vi "Callback Change Metadata.vi"(6 "Variant":variant, 8 "error in (no error)":errorcluster, 9 "Old Values":string[][](array[string]), 10 "object ref in":T1, 11 "Table Change":T2) -> (0 "error out":errorcluster)   [LabVIEW 2014, in "DAQmx Module Editor Node.lvclass"]
doc: "This VI gets called automatically when changes are made to the 'Channel Direction' column of the table and must handle changes appropriately. Register this callback using the appropriate 'Define Column' VI from the Table API."
uses:
  DAQmx Module Editor Node.lvclass
  <vilib>/NI/DCAF/Tag Editor Core/Table API/Table Manager/Cell Change.ctl
  <vilib>/NI/DCAF/Tag Editor Core/Table API/Table Manager/object ref.ctl
  <vilib>/NI/DCAF/Tag Editor Core/Configuration Editor/Classes/Engine Parent/Engine Parent Editor Node.lvclass
  <vilib>/NI/DCAF/Tag Editor Core/Configuration Editor/Classes/Module editor node/module editor node.lvclass
  module/configuration/DAQmx Module Configuration.lvclass
  module/configuration/DAQmx Module Configuration.lvclass/DAQmx Module Configuration.ctl
  <vilib>/NI/Tag Bus/tag/tag descriptor.lvclass/tag descriptor.ctl
  module/configuration/Get Line Name.vi
  <vilib>/NI/Tag Bus Module Framework/module configuration/FindDuplicate.vi
  <vilib>/Utility/error.llb/Error Cluster From Error Code.vi
  <vilib>/NI/Tag Bus Module Framework/channel/TBM channel.lvclass
  <vilib>/NI/Tag Bus/tag/tag descriptor.lvclass
  <vilib>/NI/DCAF/Tag Editor Core/Table API/Table Manager.lvlib
  <vilib>/NI/DCAF/Tag Editor Core/Table API/Table Manager/Table Manager.lvclass
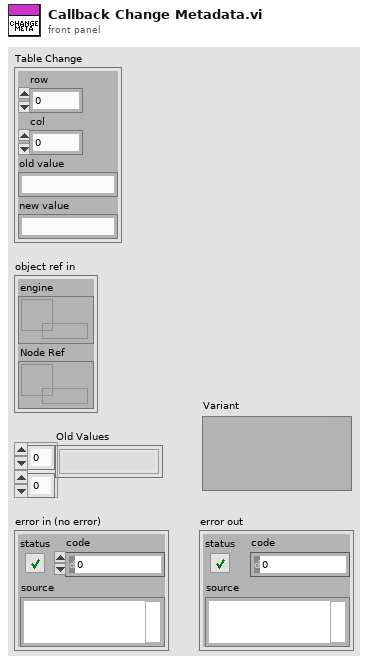
[diagram p1: front panel]
types:
  T1 = typedef "Table Manager.lvlib/Table Manager.lvclass/object ref.ctl" = cluster{"engine":refnum<data-value>, "Node Ref":refnum<data-value>}
  T2 = typedef "Table Manager.lvlib/Cell Change.ctl" = cluster{"row":i32, "col":i32, "old value":string, "new value":string}
  T3 = typedef "DAQmx Module Configuration.lvclass/Line.ctl" = cluster{"channel":refnum<class "TBM channel.lvclass">, "Physical Channel":string, "Measurement Type":T4, "Parameters":T5}
  T4 = typedef "DAQmx Module Configuration.lvclass/Measurement Type.ctl" = enum16{"Digital Input", "Digital Output", "Voltage Input", "Voltage Output", "Current Input", "Current Output", "RTD", "Thermocouple", "Strain"}
  T5 = typedef "DAQmx Module Configuration.lvclass/Parameters.ctl" = cluster{"Digital Config":cluster{"Invert Lines?":bool}, "Voltage Config":cluster{"Maximum Value (V)":dbl, "Minimum Value (V)":dbl, "in terminal configuration (V)":i32, "out terminal configuration (V)":i32}, "Current Config":cluster{"Maximum Value (A)":dbl, "Minimum Value (A)":dbl, "shunt resistor location":i32, "input terminal configuration (C)":i32, "external shunt resistor value":dbl}, "RTD Config":cluster{"Maximum Value (°C)":dbl, "Minimum Value (°C)":dbl, "resistance configuration":i32, "r0":dbl, "current excitation value":dbl, "rtd type":i32, "current excitation source":i32}, "Thermocouple Config":cluster{"Minimum Value (C)":dbl, "Maximum Value (C)":dbl, "thermocouple type":i32, "cjc source":i32, "cjc value":dbl}, "Strain Config":cluster{"Maximum Value":dbl, "Minimum Value":dbl, "bridge information":cluster{"strain configuration":i32, "lead wire resistance":dbl, "initial bridge voltage":dbl, "voltage excitation source":i32, "voltage excitation value":dbl}, "strain gage information":cluster{"gage factor":dbl, "nominal gage resistance":dbl, "poisson ratio":dbl}}}
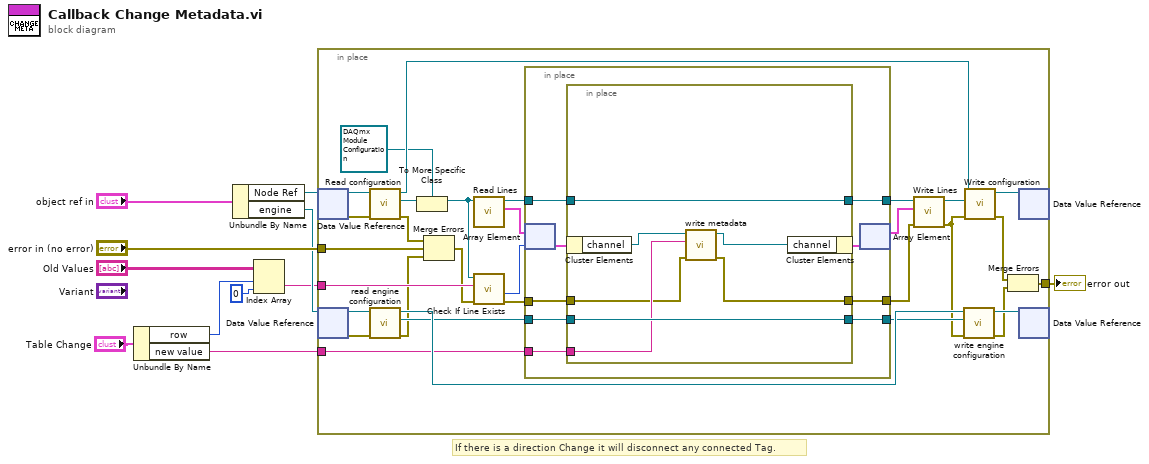
[diagram p0: block diagram]
diagram:
  # "If there is a direction Change it will disconnect any connected Tag."
  n1 = Unbundle By Name("Table Change") -> ("row"=w2:i32, "new value"=w1:string)
  n2 = Unbundle By Name("object ref in") -> ("Node Ref"=w8:refnum<data-value>, "engine"=w7:refnum<data-value>)
  n3 = Index Array(array="Old Values", index (row)=w2, index (col)=0 ("disabled index (col)")) -> (element=w3:string)
  n4 = in-place {
    in-place-border: [w35] -> w11
    in-place-border: "error in (no error)" -> [w13]
    in-place-border: w1 -> [w23]
    in-place-border: w3 -> [w22]
    n5 = in-place-dvr #1(w8) -> (w32:refnum<class "module editor node.lvclass">, w34:errorcluster)
    n6 = in-place-dvr #2(w7) -> (w41:refnum<class "Engine Parent Editor Node.lvclass">, w42:errorcluster)
    n7 = call-dynamic "Read configuration.vi"("error in"=w34, "NISE_CEF_serializable node in"=w32) -> ("error out"=w33:errorcluster, "configuration"=w30:refnum<class "NISE_CEF_serializable configuration.lvclass">, "NISE_CEF_serializable node out"=w31:refnum<class "module editor node.lvclass">)  [unwired: 7 in]
    n8 = call <vilib>:"read engine configuration.vi"("error in"=w42, "Engine Parent Editor Node in"=w41) -> ("error out"=w12:errorcluster, "engine configuration"=w19:refnum<class "engine configuration.lvclass">, "Engine Parent Editor Node out"=w38:refnum<class "Engine Parent Editor Node.lvclass">)  [unwired: 7 in]
    n9 = To More Specific Class(target class=refnum<class "DAQmx Module Configuration.lvclass"> refnum ("tag bus configurable plugin module configuration"), reference=w30) -> (specific class reference=w27:refnum<class "DAQmx Module Configuration.lvclass">)  [unwired: 1 in, 1 out]
    n10 = Merge Errors(w33, w13, w12) -> (w17:errorcluster)
    n11 = call "Read Lines.vi"("Daqmx Module configuration in"=w27) -> ("Lines"=w26:T3[], "Daqmx Module configuration out"=w21:refnum<class "DAQmx Module Configuration.lvclass">)  [unwired: 8 in, 1 out]
    n12 = call-dynamic "Check If Line Exists.vi"("error in"=w17, "Name to Locate"=w22, "Daqmx Module configuration in"=w27) -> ("error out"=w16:errorcluster, "Index"=w24:i32)  [unwired: 4 in, 3 out]
    n13 = in-place {
      in-place-border: w23 -> [w49]
      in-place-border: w21 -> [w48]
      in-place-border: [w47] -> w20
      in-place-border: w19 -> [w46]
      in-place-border: [w45] -> w18
      in-place-border: w16 -> [w44]
      in-place-border: [w43] -> w15
      n14 = in-place-array #3(w26, w24) -> (w51:T3)
      n15 = in-place {
        in-place-border: w49 -> [w54]
        in-place-border: w48 -> [w58]
        in-place-border: [w58] -> w47
        in-place-border: w46 -> [w57]
        in-place-border: [w57] -> w45
        in-place-border: w44 -> [w53]
        in-place-border: [w52] -> w43
        n16 = in-place-cluster #4(w51) -> ("channel"=w56:refnum<class "TBM channel.lvclass">)
        n17 = call <vilib>:"write metadata.vi"("error in"=w53, "metadata"=w54, "system tag in"=w56) -> ("error out"=w52:errorcluster, "system tag out"=w55:refnum<class "TBM channel.lvclass">)  [unwired: 7 in]
        n18 = in-place-cluster #4("channel"=w55) -> (w50:T3)
      }
      n19 = in-place-array #3(w50) -> (w25:T3[])  [unwired: 1 out]
    }
    n20 = call "Write Lines.vi"("error in (no error)"=w15, "Lines"=w25, "Daqmx Module configuration in"=w20) -> ("error out"=w14:errorcluster, "Daqmx Module configuration out"=w28:refnum<class "DAQmx Module Configuration.lvclass">)  [unwired: 7 in]
    n21 = call <vilib>:"write engine configuration.vi"("error in"=w14, "engine configuration"=w18, "Engine Parent Editor Node in"=w38) -> ("error out"=w37:errorcluster, "Engine Parent Editor Node out"=w40:refnum<class "Engine Parent Editor Node.lvclass">)  [unwired: 7 in]
    n22 = call-dynamic "Write configuration.vi"("error in"=w14, "configuration"=w28, "NISE_CEF_serializable node in"=w31) -> ("error out"=w36:errorcluster, "NISE_CEF_serializable node out"=w39:refnum<class "module editor node.lvclass">)  [unwired: 7 in]
    n23 = Merge Errors(w36, w37) -> (w35:errorcluster)
    n24 = in-place-dvr #1(w39) -> ()  [unwired: 2 out]
    n25 = in-place-dvr #2(w40) -> ()  [unwired: 2 out]
  }
  "error out" <- w11
